vi "Acel_calib_noise_files_out.vi"(9 "Pattern frequency (Hz)":dbl, 10 "Frecuencia\nmuestreo":dbl, 11 "Acel Cal measurements in":sgl[][](array[numeric])) -> (0 "Measurements OK":bool, 2 "Reporting 3":string, 3 "Acel Cal measurements out 2":sgl[][](array[numeric]))   [LabVIEW 2015]
uses:
  <vilib>/Analysis/5stat.llb/RMS (DBL).vi
  <vilib>/measure/madcrms.llb/Basic Averaged DC-RMS for 1 Chan.vi
  <vilib>/measure/NI_MAPro.lvlib
  <vilib>/Analysis/NI_AALPro.lvlib
  <vilib>/Analysis/NI_AALBase.lvlib
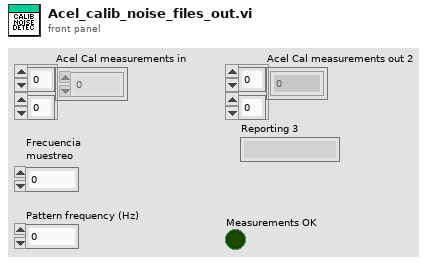
[diagram p1: front panel]
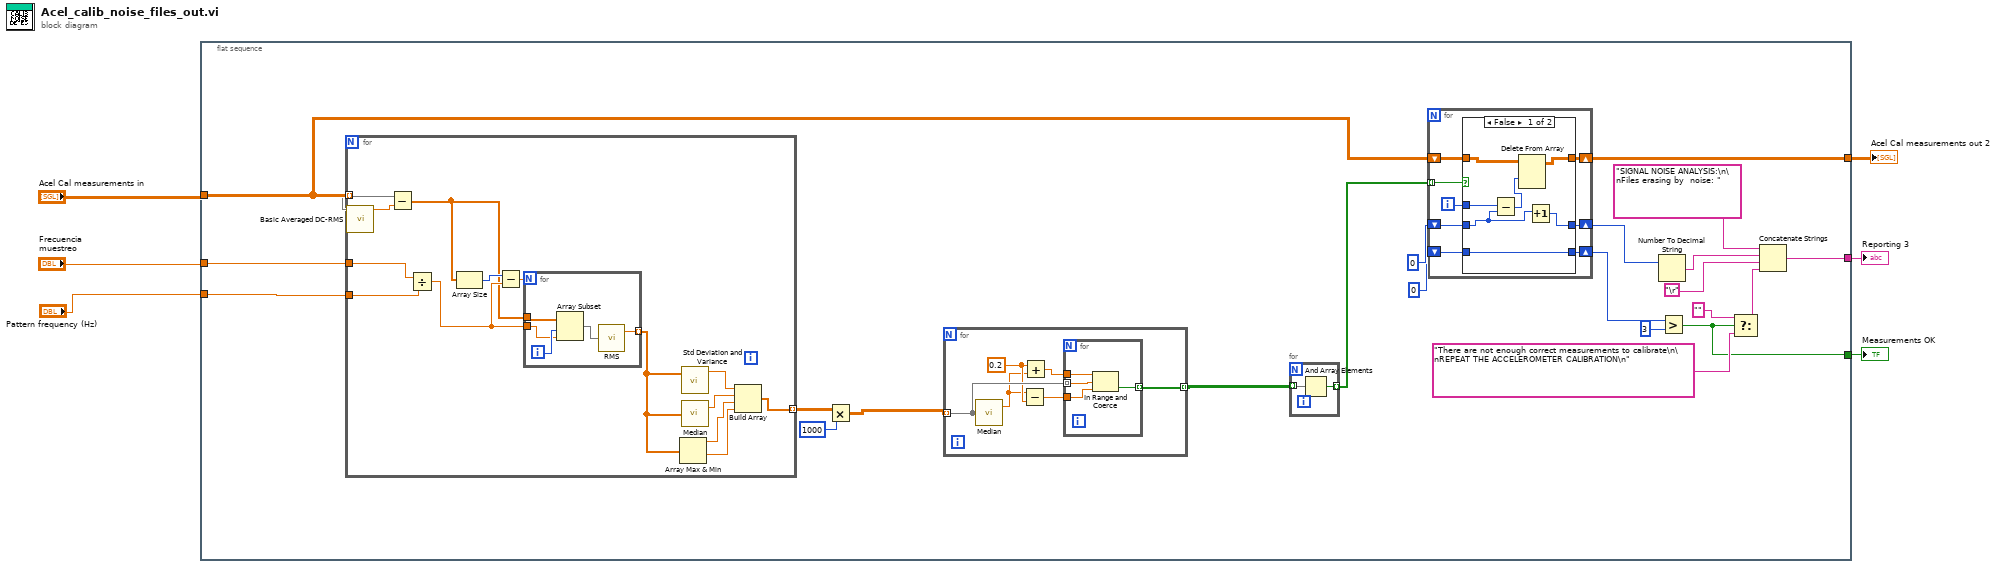
[diagram p0: block diagram]
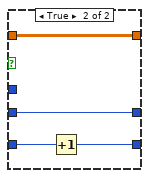
[diagram p2: hidden frame]
diagram:
  n1 = flat-sequence {
    tunnel: "Acel Cal measurements in" -> [w7]
    tunnel: [w24] -> w3
    tunnel: "Frecuencia\nmuestreo" -> [w23]
    tunnel: "Pattern frequency (Hz)" -> [w22]
    tunnel: [w11] -> w2
    tunnel: [w10] -> w1
    frame #0 {
      n2 = for {
        tunnel: w7 -> [w72] mode=indexing
        tunnel: [w65] -> w28 mode=indexing
        tunnel: w23 -> [w60]
        tunnel: w22 -> [w61]
        n3 = call-poly <vilib>:"Basic Averaged DC-RMS.vi"("signal in"=w72) -> ("DC value"=w73:dbl)  [unwired: 7 in, 3 out]
        n4 = Subtract(x=w72, y=w73) -> (x-y=w62:dbl[])
        n5 = Divide(x=w60, y=w61) -> (x/y=w69:dbl)
        n6 = Array Size(array=w62) -> (size(s)=w70:i32)
        n7 = Subtract(x=w70, y=w69) -> (x-y=w71:dbl)
        n8 = for {
          N: w71 -> [_]
          tunnel: w69 -> [w75]
          tunnel: [w78] -> w63 mode=indexing
          tunnel: w62 -> [w77]
          i -> [w76]
          n9 = Array Subset(array=w77, index=w76, length=w75) -> (w74:dbl[])
          n10 = call-poly <vilib>:"RMS.vi"("X"=w74) -> ("rms value"=w78:dbl)  [unwired: 1 out]
        }
        n11 = Array Max & Min(array=w63) -> (max value=w67:dbl, min value=w66:dbl)  [unwired: 2 out]
        n12 = call <vilib>:"Std Deviation and Variance.vi"("X"=w63) -> ("mean"=w64:dbl)  [unwired: 1 in, 2 out]
        n13 = call <vilib>:"Median.vi"("X"=w63) -> ("median"=w68:dbl)  [unwired: 1 out]
        n14 = Build Array(w64, w68, w67, w66) -> (w65:dbl[])
      }
      n15 = Multiply(x=w28, y=1000 ("median")) -> (x*y=w9:dbl[][])
      n16 = for {
        tunnel: w9 -> [w55] mode=indexing
        tunnel: [w50] -> w8 mode=indexing
        w53 = 0.2 ("x")
        n17 = call <vilib>:"Median.vi"("X"=w55) -> ("median"=w51:dbl)  [unwired: 1 out]
        n18 = Subtract(x=w51, y=w53) -> (x-y=w52:dbl)
        n19 = Add(x=w53, y=w51) -> (x+y=w54:dbl)
        n20 = for {
          tunnel: w55 -> [w59] mode=indexing
          tunnel: w54 -> [w58]
          tunnel: w52 -> [w57]
          tunnel: [w56] -> w50 mode=indexing
          n21 = In Range and Coerce(upper limit=w58, x=w59, lower limit=w57) -> (In Range?=w56:bool)  [unwired: 1 out]
        }
      }
      n22 = for {
        tunnel: w8 -> [w49] mode=indexing
        tunnel: [w48] -> w25 mode=indexing
        n23 = And Array Elements(Boolean array=w49) -> (logical AND=w48:bool)
      }
      n24 = for {
        shift-right: [w35] -> w24
        shift-left: w7 -> [w36]
        tunnel: w25 -> [w34] mode=indexing
        shift-right: [w31] -> w21
        shift-left: 0 ("index of element") -> [w32]
        shift-right: [w29] -> w16
        shift-left: 0 ("index of element") -> [w30]
        i -> [w33]
        n25 = case shown="False" w34 {
          tunnel: w36 -> [w43 w47]
          tunnel: [w42 w47] -> w35
          tunnel: w33 -> [w41 _]
          tunnel: w32 -> [w40 w46]
          tunnel: [w39 w46] -> w31
          tunnel: w30 -> [w37 w45]
          tunnel: [w37 w44] -> w29
          frame False {
            n26 = Subtract(x=w41, y=w40) -> (x-y=w38:i32)
            n27 = Delete From Array(array=w43, index (row)=w38) -> (array with subset deleted=w42:sgl[][])  [unwired: 2 in, 1 out]
            n28 = Increment(x=w40) -> (x+1=w39:i32)
          }
          frame True {
            n29 = Increment(x=w45) -> (x+1=w44:i32)
          }
        }
      }
      n30 = Number To Decimal String(number=w21) -> (decimal integer string=w19:string)  [unwired: 1 in]
      n31 = Greater?(x=w16, y=3) -> (0:w10:bool)
      n32 = Select(t="", s=w10, f="There are not enough correct measurements to calibrate\n\nREPEAT THE ACCELEROMETER CALIBRATION\n") -> (s? t:f=w12:string)
      n33 = Concatenate Strings("SIGNAL NOISE ANALYSIS:\n\nFiles erasing by  noise: ", w19, "\r", w12) -> (w11:string)
    }
  }
  "Acel Cal measurements out 2" <- w3
  "Reporting 3" <- w2
  "Measurements OK" <- w1
